vi "GOOP_XControl_Item_OnPopUpMenu.vi"(11 "Object":u64) -> ()   [LabVIEW 2012]
uses:
  <resource>/Framework/Providers/API/mxLvMenuItem.ctl
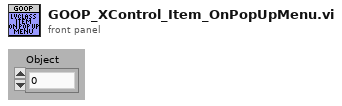
[diagram p1: front panel]
types:
  T1 = typedef "mxLvMenuItem.ctl" = cluster{"Menu Name":string, "Description":string, "Icon File Name":path, "Menu Tag":string, "Enabled":bool, "Checked":bool, "Separator":bool, "Batchable":bool, "Weight":i32, "Batch Mode (Ignored if Not Batchable)":enum32{"Show If All Items Support Command", "Show If Any Items Support Command"}, "Menu Location":enum32{"<None>", "Project", "Project / Build Specifications", "Tools", "Tools / Source Control", "Tools / Real-Time Module", "Help"}, "Exclude From Getting Started Window Menu":bool}
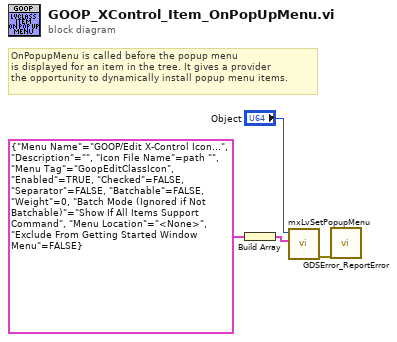
[diagram p0: block diagram]
diagram:
  # "OnPopupMenu is called before the popup menu\nis displayed for an item in the tree. It gives a provider\nthe opportunity to dynamically install popup menu items."
  n1 = Build Array(T1 {"Menu Name"="GOOP/Edit X-Control Icon...", "Description"="", "Icon File Name"=path "", "Menu Tag"="GoopEditClassIcon", "Enabled"=TRUE, "Checked"=FALSE, "Separator"=FALSE, "Batchable"=FALSE, "Weight"=0, "Batch Mode (Ignored if Not Batchable)"=enum."Show If All Items Support Command", "Menu Location"=enum."<None>", "Exclude From Getting Started Window Menu"=FALSE} ("Menu Item")) -> (w3:T1[])
  n2 = call <resource>:"mxLvSetPopupMenu.vi"("Popup Menu Items"=w3, "Item"="Object") -> ("error out"=w2:errorcluster)  [unwired: 8 in, 1 out]
  n3 = call <resource>:"GDSError_ReportError.vi"("error in (no error)"=w2) -> ()  [unwired: 18 in, 1 out]
